vi "Child_Create.vi"(0 "reference in":refnum<class "Child.lvclass">, 5 "error in (no error)":errorcluster) -> (14 "reference out":refnum<class "Child.lvclass">, 19 "error out":errorcluster)   [LabVIEW 2019, in "Child.lvclass"]
uses:
  Child.lvclass
  C:/Users/Tiba/Desktop/TCSS OOP/Class/Parent_class/Parent.lvclass
  Parent_class/Parent.lvclass
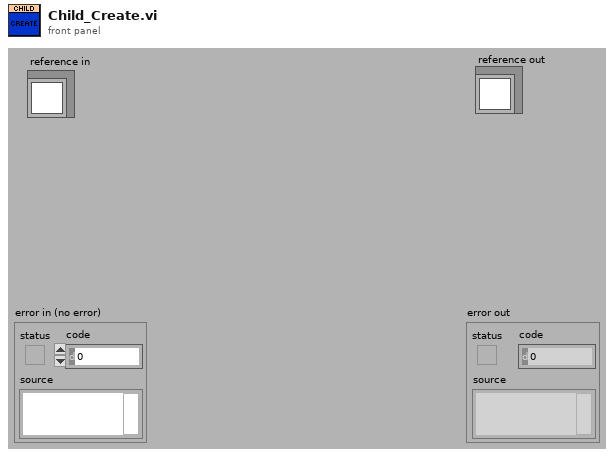
[diagram p1: front panel]
types:
  T1 = typedef "Child.lvclass/ObjectAttributes.ctl" = cluster{"Attribute0":dbl}
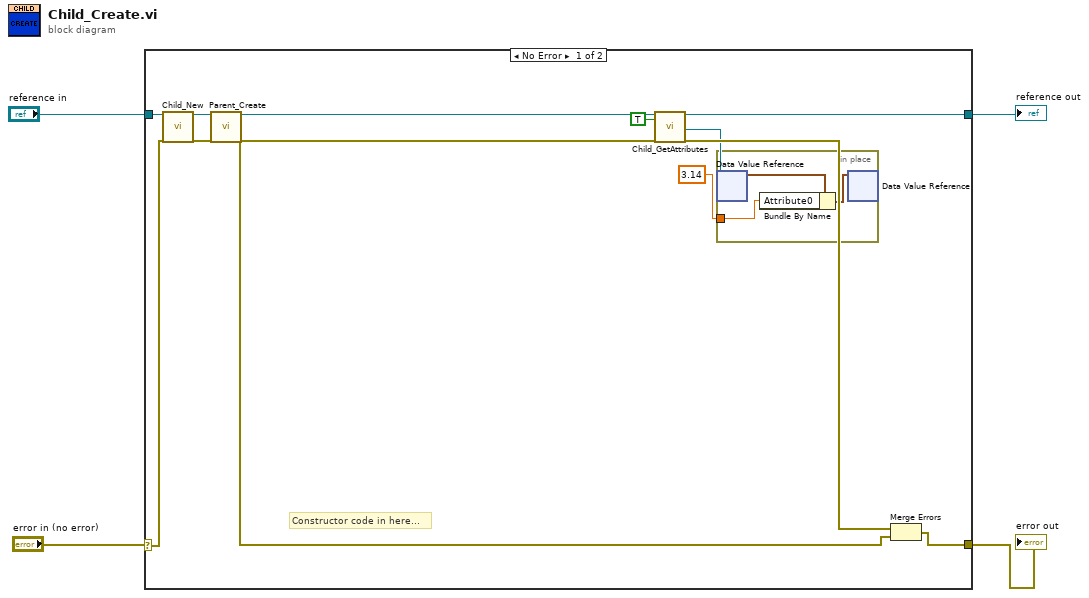
[diagram p0: block diagram]
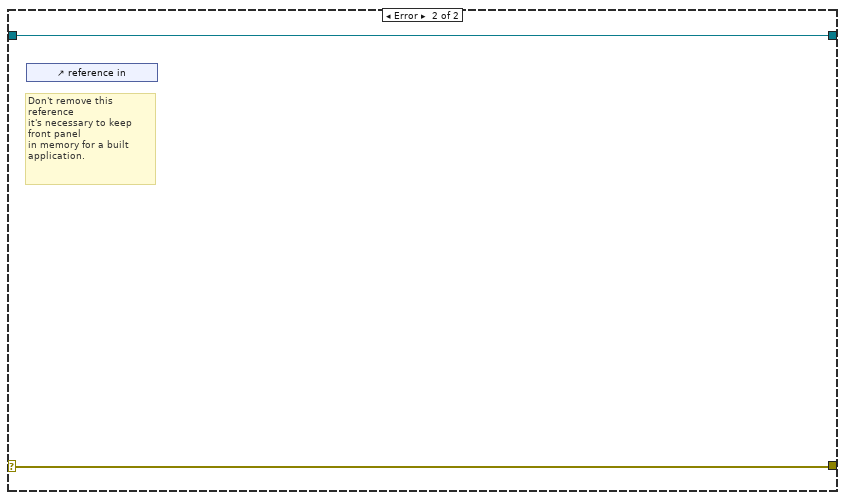
[diagram p2: hidden frame]
diagram:
  n1 = case shown="No Error" "error in (no error)" {
    selector: "error in (no error)" -> [w10 w21]
    tunnel: [w14 w21] -> w4
    tunnel: "reference in" -> [w11 w20]
    tunnel: [w16 w20] -> w2
    frame No Error {
      # "Constructor code in here..."
      n2 = call "Child_New.vi"("reference in"=w11, "error in (no error)"=w10) -> ("reference out"=w9:refnum<class "Child.lvclass">, "error out"=w8:errorcluster)  [unwired: 14 in, 2 out]
      n3 = call "Parent_Create.vi"("reference in"=w9, "error in (no error)"=w8) -> ("reference out"=w15:refnum<class "Child.lvclass">, "error out"=w12:errorcluster)  [unwired: 16 in]
      n4 = call "Child_GetAttributes.vi"("reference in"=w15, "OnlyGetDvrReference(False)"=TRUE, "error in (no error)"=w12) -> ("reference out"=w16:refnum<class "Child.lvclass">, "DataRef"=w6:refnum<data-value>, "error out"=w13:errorcluster)  [unwired: 13 in, 1 out]
      n5 = in-place {
        in-place-border: 3.14 ("attribute1") -> [w18]
        n6 = in-place-dvr #1(w6) -> (w19:T1)  [unwired: 1 out]
        n7 = Bundle By Name(cluster=w19, "Attribute0"=w18) -> (w17:T1)
        n8 = in-place-dvr #1(w17) -> ()  [unwired: 2 out]
      }
      n9 = Merge Errors(w13, w12) -> (w14:errorcluster)
    }
    frame Error {
      # "Don't remove this reference\nit's necessary to keep front panel\nin memory for a built application."
      n10 = control-ref of="reference in"() -> ()  [unwired: 1 out]
    }
  }
  "error out" <- w4
  "reference out" <- w2
